vi "gentec-M-Link.Close Connection.vi"(0 "VISA resource In":refnum<visa-resource-name>, 5 "error in (no error)":errorcluster) -> (19 "error out":errorcluster)   [LabVIEW 2014, in "gentec-M-Link - Driver.lvlib"]
doc: "This VI closes a VISA connection."
uses:
  gentec-M-Link - Driver.lvlib
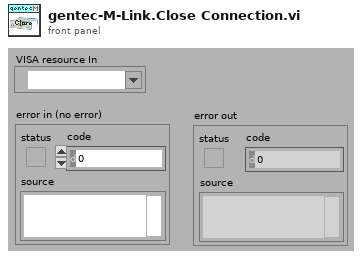
[diagram p1: front panel]
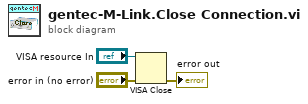
[diagram p0: block diagram]
diagram:
  n1 = VISA Close(VISA resource name="VISA resource In", error in (no error)="error in (no error)") -> (error out=→"error out":errorcluster)
